vi "POST.vi"(8 "error in":errorcluster, 10 "httpRequest":refnum<class "httpRequest.lvclass">, 11 "http-client in":refnum<class "httpClient.lvclass">) -> (0 "error out":errorcluster, 2 "httpResponse":refnum<class "httpResponse.lvclass">, 3 "http-client out":refnum<class "httpClient.lvclass">)   [LabVIEW 2020, in "httpClient.lvlib" / "httpClient.lvclass"]
uses:
  httpClient.lvclass
  httpRequest/httpRequest.lvclass
  httpResponse/httpResponse.lvclass
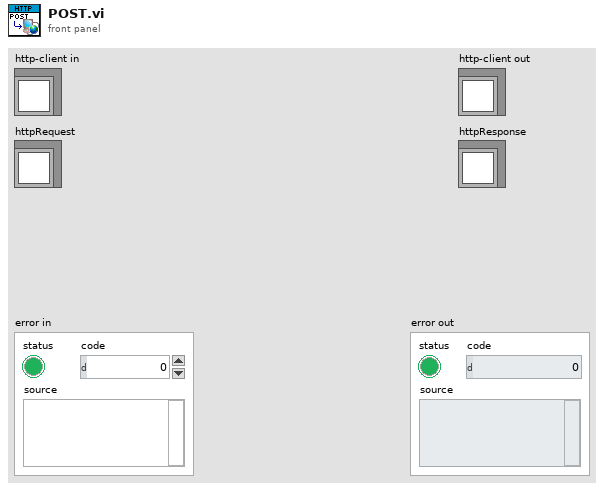
[diagram p1: front panel]
types:
  T1 = typedef "httpClient.lvlib/httpRequest.lvclass/Multipart data -- cluster.ctl" = cluster{"Name":string, "Value":string, "File":path, "Filename":string, "MIME type":string}
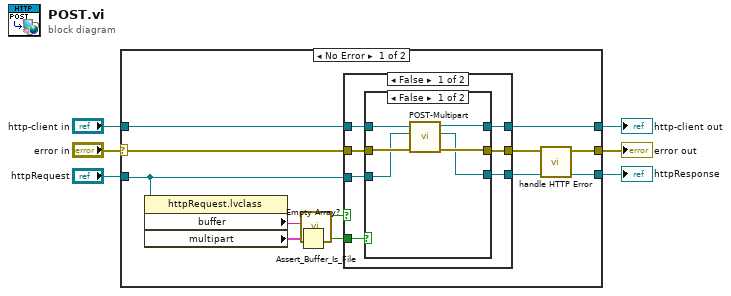
[diagram p0: block diagram]
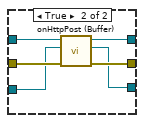
[diagram p2: hidden frame]
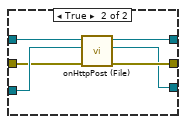
[diagram p3: hidden frame]
diagram:
  n1 = case shown="No Error" "error in" {
    selector: "error in" -> [w15 w45]
    tunnel: [w13 w45] -> w5
    tunnel: [w16 w44] -> w3
    tunnel: "http-client in" -> [w17 w44]
    tunnel: [w7 _] -> w2
    tunnel: "httpRequest" -> [w11 _]
    frame No Error {
      n2 = property class="httpRequest.lvclass"(reference=w11) -> ("buffer"=w12:string, "multipart"=w10:T1[])  [unwired: 1 in, 2 out]
      n3 = Empty Array?(array=w10) -> (empty?=w9:bool)
      n4 = call "Assert_Buffer_Is_File.vi"("buffer"=w12) -> ("is File?"=w18:bool)  [unwired: 9 in, 1 out]
      n5 = case shown="False" w18 {
        tunnel: w17 -> [w25 w43]
        tunnel: [w21 w42] -> w16
        tunnel: [w20 w38] -> w8
        tunnel: w11 -> [w23 w41]
        tunnel: [w22 w40] -> w14
        tunnel: w15 -> [w24 w39]
        tunnel: w9 -> [w19 _]
        frame False {
          n6 = case shown="False" w19 {
            tunnel: w25 -> [w31 w37]
            tunnel: w24 -> [w29 w36]
            tunnel: w23 -> [w27 w35]
            tunnel: [w28 w34] -> w22
            tunnel: [w30 w33] -> w21
            tunnel: [w26 w32] -> w20
            frame False {
              n7 = call "POST-Multipart.vi"("error in"=w29, "httpRequest"=w27, "http-client in"=w31) -> ("error out"=w28:errorcluster, "httpResponse"=w26:refnum<class "httpResponse.lvclass">, "http-client out"=w30:refnum<class "httpClient.lvclass">)  [unwired: 6 in]
            }
            frame True {
              n8 = call-dynamic "onHttpPost (Buffer).vi"("error in"=w36, "httpRequest"=w35, "http-method in"=w37) -> ("error out"=w34:errorcluster, "httpResponse"=w32:refnum<class "httpResponse.lvclass">, "http-method out"=w33:refnum<class "httpClient.lvclass">)  [unwired: 6 in]
            }
          }
        }
        frame True {
          n9 = call-dynamic "onHttpPost (File).vi"("error in"=w39, "httpRequest"=w41, "http-method in"=w43) -> ("error out"=w40:errorcluster, "httpResponse"=w38:refnum<class "httpResponse.lvclass">, "http-method out"=w42:refnum<class "httpClient.lvclass">)  [unwired: 6 in]
        }
      }
      n10 = call "handle HTTP Error.vi"("httpResponse"=w8, "error in (no error)"=w14) -> ("httpResponse out"=w7:refnum<class "httpResponse.lvclass">, "error out"=w13:errorcluster)  [unwired: 8 in]
    }
    frame Error {
    }
  }
  "error out" <- w5
  "http-client out" <- w3
  "httpResponse" <- w2
